vi "Get Status.vi"(8 "error in (no error)":errorcluster, 11 "arm motor_EtherCAT in":refnum<class "NI_Robotics_KUKA youBot Arm Motor_EtherCAT.lvclass">) -> (0 "error out":errorcluster, 2 "status flag":T1, 3 "arm motor_EtherCAT out":refnum<class "NI_Robotics_KUKA youBot Arm Motor_EtherCAT.lvclass">)   [LabVIEW 2017, in "NI_Robotics_KUKA youBot Host.lvlib" / "NI_Robotics_KUKA youBot Arm Motor_EtherCAT.lvclass"]
uses:
  <vilib>/robotics/KUKA youBot/Motor/Arm Motor EtherCAT/NI_Robotics_KUKA youBot Arm Motor_EtherCAT.lvclass
  <vilib>/robotics/KUKA youBot/EtherCAT/CmdCtrls/Error_Status Flag.ctl
  <vilib>/robotics/KUKA youBot/Motor/Arm Motor EtherCAT/NI_Robotics_KUKA youBot Arm Motor_EtherCAT.lvclass/NI_Robotics_KUKA youBot Arm Motor_EtherCAT.ctl
  <vilib>/robotics/KUKA youBot/NI_Robotics_KUKA youBot Host.lvlib
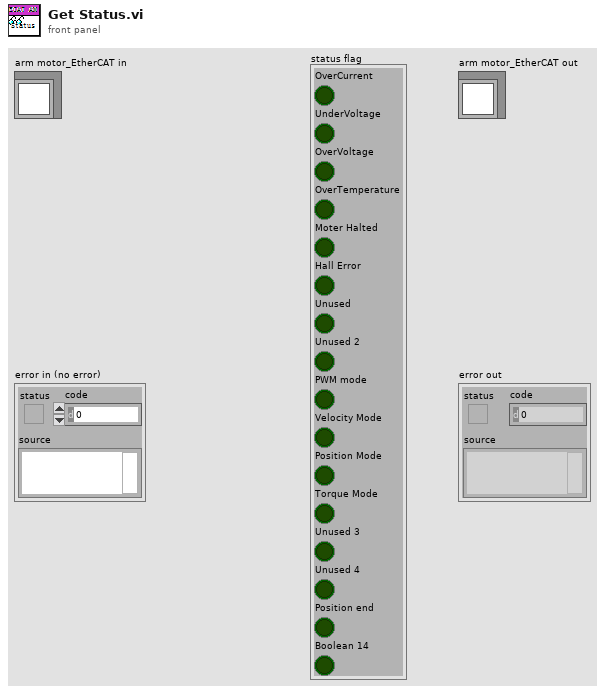
[diagram p1: front panel]
types:
  T1 = typedef "NI_Robotics_KUKA youBot Host.lvlib/Error_Status Flag.ctl" = cluster{"OverCurrent":bool, "UnderVoltage":bool, "OverVoltage":bool, "OverTemperature":bool, "Moter Halted":bool, "Hall Error":bool, "Unused":bool, "Unused 2":bool, "PWM mode":bool, "Velocity Mode":bool, "Position Mode":bool, "Torque Mode":bool, "Unused 3":bool, "Unused 4":bool, "Position end":bool, "Boolean 14":bool}
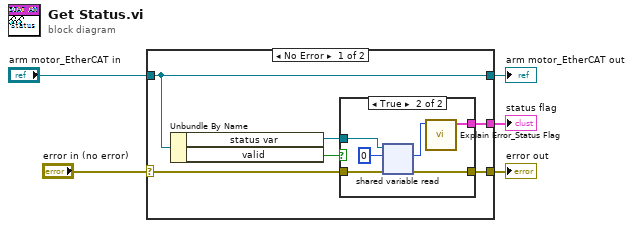
[diagram p0: block diagram]
diagram:
  n1 = case shown="No Error" "error in (no error)" {
    selector: "error in (no error)" -> [w9 w19]
    tunnel: [w8 w19] -> w4
    tunnel: [w11 w20] -> w2
    tunnel: "arm motor_EtherCAT in" -> [w11 w20]
    tunnel: [w6 _] -> w1
    frame No Error {
      n2 = Unbundle By Name(w11) -> ("status var"=w7:refnum<k21>, "valid"=w10:bool)
      n3 = case shown="True" w10 {
        tunnel: w9 -> [w12 w18]
        tunnel: [w12 w17] -> w8
        tunnel: w7 -> [_ w16]
        tunnel: [_ w13] -> w6
        frame False {
        }
        frame True {
          n4 = shared-variable-read(w16, w18, i16 0) -> (w17:errorcluster, w14:i16)  [unwired: 2 out]
          n5 = call <vilib>:"Explain Error_Status Flag.vi"("Error/Status Flag"=w14) -> ("Expalined Flag"=w13:T1)  [unwired: 10 in]
        }
      }
    }
    frame Error {
    }
  }
  "error out" <- w4
  "arm motor_EtherCAT out" <- w2
  "status flag" <- w1
